vi "电机参数.vi"() -> (0 "参数输出":T1)   [LabVIEW 2014]
panel:
  in  "Stop Button":bool
  in  "Lq":dbl
  in  "Ld":dbl
  in  "转子漏感":dbl
  in  "定子漏感":dbl
  in  "励磁电感":dbl
  in  "转子电阻（欧）":dbl
  in  "定子电阻（欧）":dbl
  in  "电机类型":enum16{"异步电机", "永磁同步电机"}(ring)
  in  "逆变器直流电压（Vdc）":dbl
  in  "电机最大转矩（Nm）":dbl
  in  "电机最大转速（rpm）":dbl
  in  "电机极对数":u32
  in  "电机额定功率（kW）":dbl
  in  "电机额定转速（rpm）":dbl
  in  "电机额定电流（有效值 A）":dbl
  in  "电机额定电压（有效值 V）":dbl
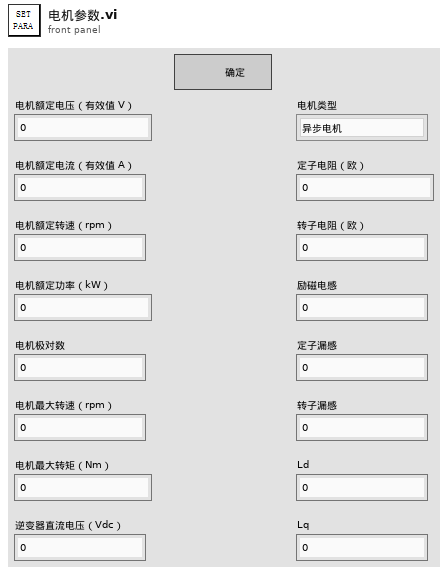
[diagram p1: front panel]
types:
  T1 = cluster{"电机额定电压（有效值 V）":dbl, "电机额定电流（有效值 A）":dbl, "电机额定转速（rpm）":dbl, "电机额定功率（kW）":dbl, "电机极对数":u32, "电机最大转速（rpm）":dbl, "电机最大转矩（Nm）":dbl, "逆变器直流电压（Vdc）":dbl, "电机类型":enum16{"异步电机", "永磁同步电机"}, "定子电阻（欧）":dbl, "转子电阻（欧）":dbl, "励磁电感":dbl, "定子漏感":dbl, "转子漏感":dbl, "Ld":dbl, "Lq":dbl}
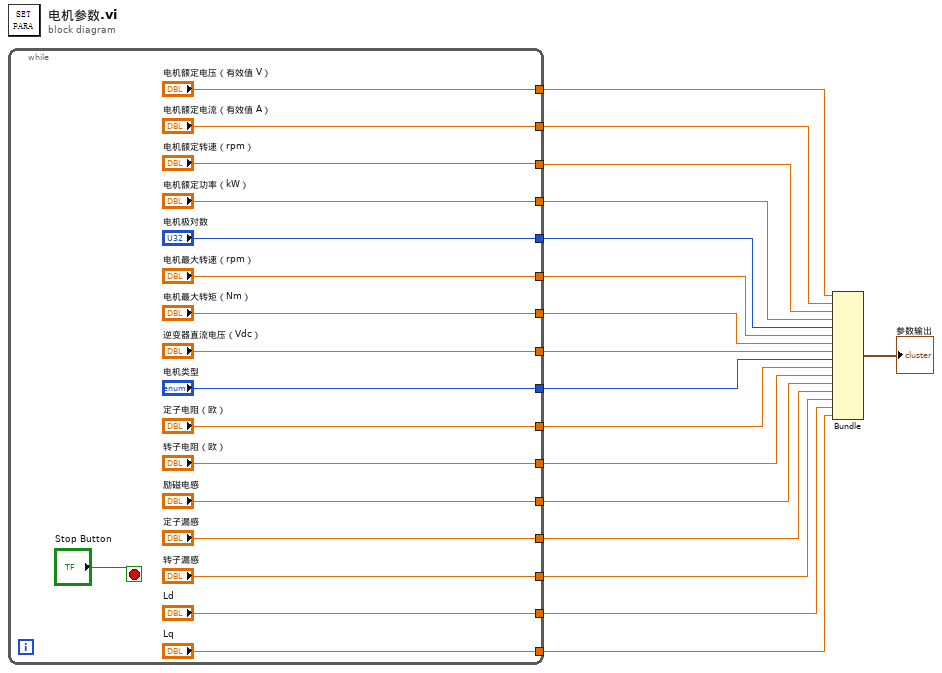
[diagram p0: block diagram]
diagram:
  n1 = while {
    tunnel: ["电机额定电压（有效值 V）"] -> w17
    tunnel: ["电机额定电流（有效值 A）"] -> w16
    tunnel: ["电机额定转速（rpm）"] -> w15
    tunnel: ["电机额定功率（kW）"] -> w14
    tunnel: ["电机极对数"] -> w13
    tunnel: ["电机最大转速（rpm）"] -> w12
    tunnel: ["电机最大转矩（Nm）"] -> w11
    tunnel: ["逆变器直流电压（Vdc）"] -> w10
    tunnel: ["电机类型"] -> w9
    tunnel: ["定子电阻（欧）"] -> w8
    tunnel: ["转子电阻（欧）"] -> w7
    tunnel: ["励磁电感"] -> w6
    tunnel: ["定子漏感"] -> w5
    tunnel: ["转子漏感"] -> w4
    tunnel: ["Ld"] -> w3
    tunnel: ["Lq"] -> w2
    stop <- "Stop Button" stop-if-true
  }
  n2 = Bundle("电机额定电压（有效值 V）"=w17, "电机额定电流（有效值 A）"=w16, "电机额定转速（rpm）"=w15, "电机额定功率（kW）"=w14, "电机极对数"=w13, "电机最大转速（rpm）"=w12, "电机最大转矩（Nm）"=w11, "逆变器直流电压（Vdc）"=w10, "电机类型"=w9, "定子电阻（欧）"=w8, "转子电阻（欧）"=w7, "励磁电感"=w6, "定子漏感"=w5, "转子漏感"=w4, "Ld"=w3, "Lq"=w2) -> (→"参数输出":T1)  [unwired: 1 in]
